vi "111-Main.vi"() -> ()   [LabVIEW 2020]
panel:
  in  "振动判定":T1={"频率检测段1振幅"={"单位"="dB", "下限"=0.0, "上限"=50.0}, "频率检测段2振幅"={"单位"="dB", "下限"=0.0, "上限"=40.0}, "频率检测段3振幅"={"单位"="dB", "下限"=0.0, "上限"=40.0}, "频率检测段4振幅"={"单位"="dB", "下限"=0.0, "上限"=40.0}, "频率检测段5振幅"={"单位"="dB", "下限"=0.0, "上限"=40.0}}
  out "字符串 8":string
  out "字符串 7":string
  out "字符串 6":string
  out "字符串 5":string
  out "字符串 4":string
  out "字符串 3":string
  out "字符串 2":string
  out "字符串":string
  in  "表格控件":string[][](table)
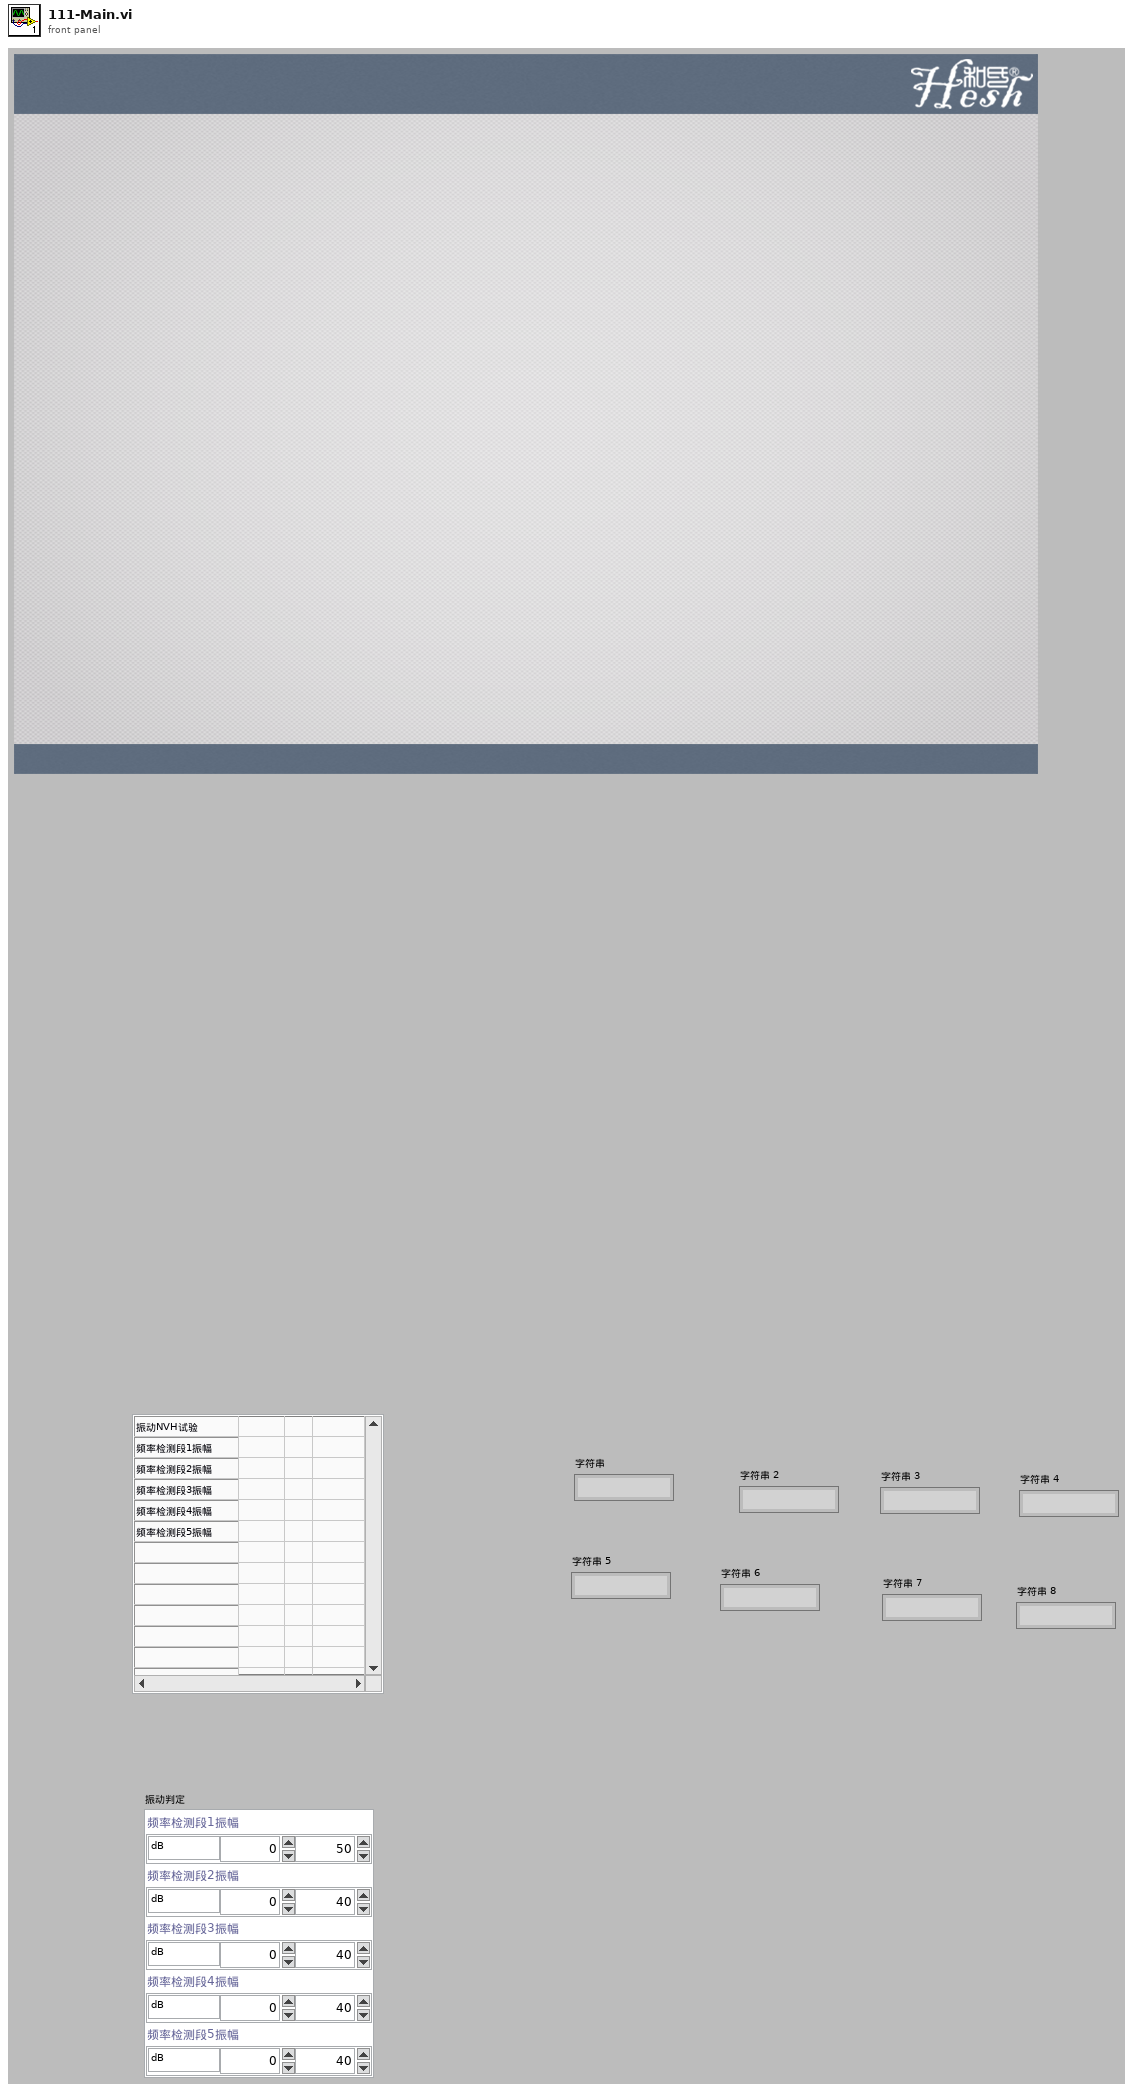
[diagram p1: front panel]
types:
  T1 = cluster{"频率检测段1振幅":cluster{"单位":string, "下限":dbl, "上限":dbl}, "频率检测段2振幅":cluster{"单位":string, "下限":dbl, "上限":dbl}, "频率检测段3振幅":cluster{"单位":string, "下限":dbl, "上限":dbl}, "频率检测段4振幅":cluster{"单位":string, "下限":dbl, "上限":dbl}, "频率检测段5振幅":cluster{"单位":string, "下限":dbl, "上限":dbl}}
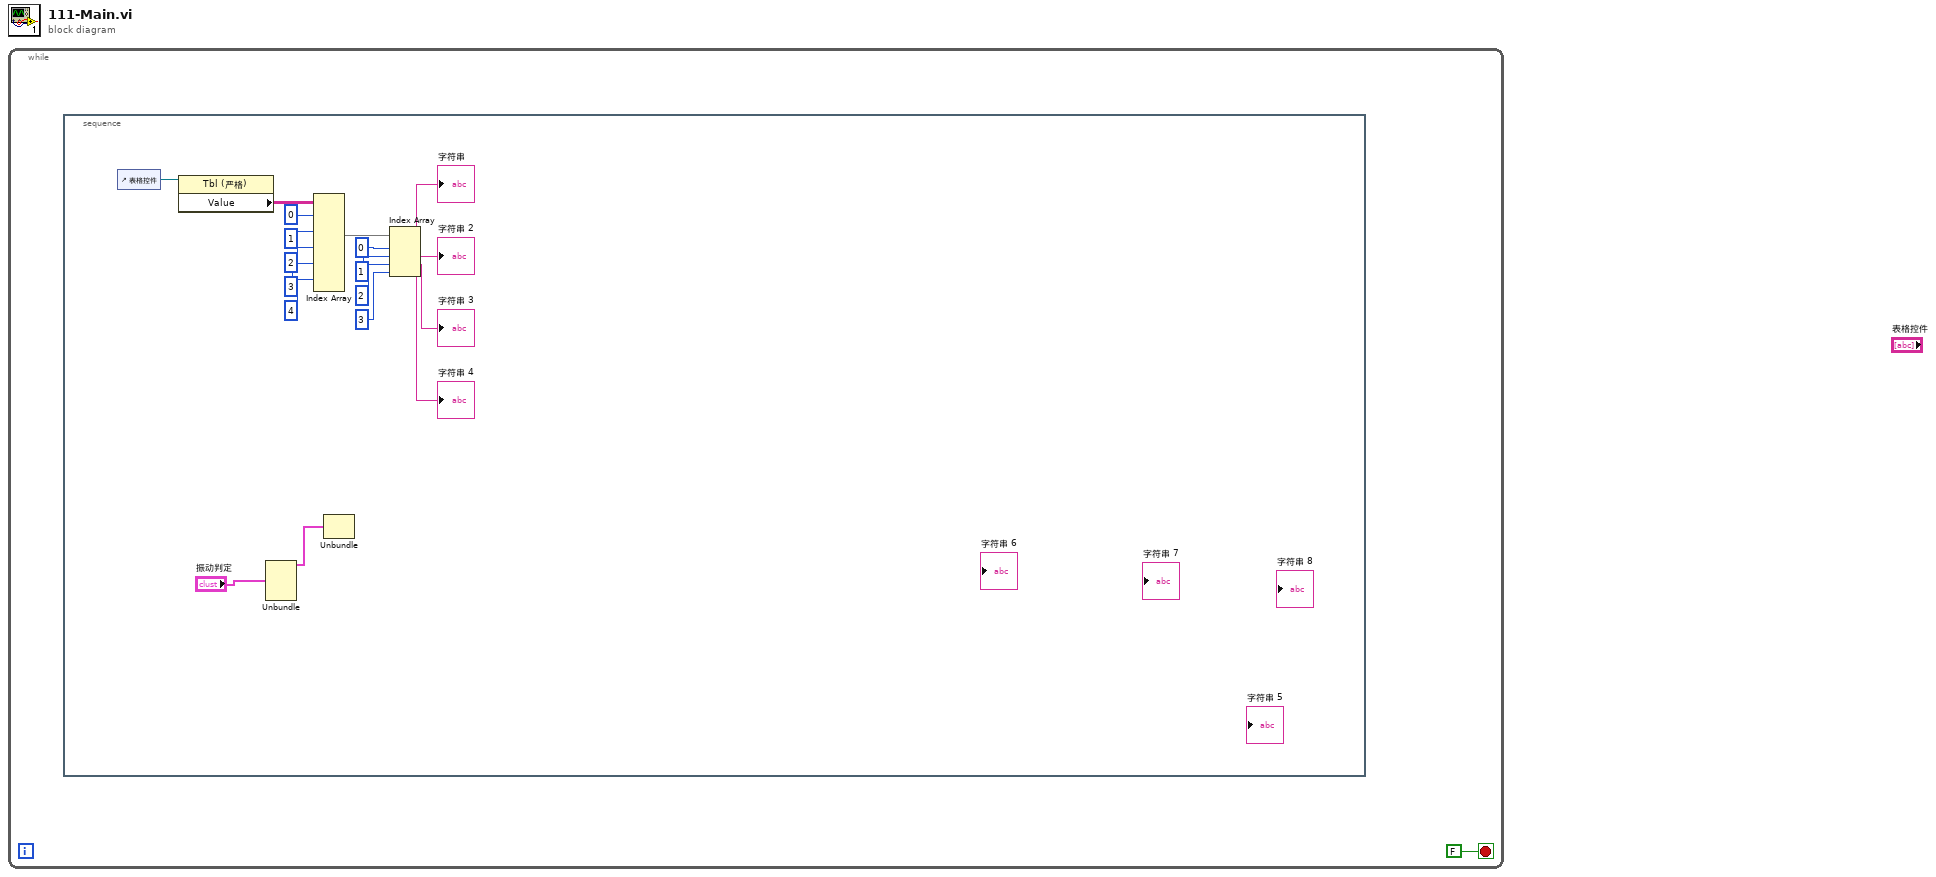
[diagram p0: block diagram]
diagram:
  n1 = while {
    stop <- FALSE stop-if-true
    n2 = stacked-sequence {
      frame #0 {
        n3 = control-ref of="表格控件"() -> (w19:refnum<vi>)
        n4 = property class="Tbl (严格)"(reference=w19) -> ("Value"=w18:string[][])  [unwired: 1 in, 2 out]
        n5 = Unbundle("振动判定") -> ("频率检测段1振幅"=w2:cluster{"单位":string, "下限":dbl, "上限":dbl})  [unwired: 4 out]
        n6 = Index Array(array=w18, index (row) #1=0 ("索引 (行)"), index (row) #2=1 ("索引 (行)"), index (row) #3=2 ("索引 (行)"), index (row) #4=3 ("禁用的索引 (列)"), index (row) #5=4 ("索引 (列)")) -> (element #2=w4:string[])  [unwired: 5 in, 4 out]
        n7 = Unbundle(w2) -> ()  [unwired: 3 out]
        n8 = Index Array(array=w4, index #1=0 ("索引 (行)"), index #2=1 ("索引 (行)"), index #3=2 ("索引 (行)"), index #4=3 ("禁用的索引 (列)")) -> (element #1=→"字符串":string, element #2=→"字符串 2":string, element #3=→"字符串 3":string, element #4=→"字符串 4":string)
      }
    }
  }
